vi "ResponseStringToSignalCluster(obj).vi"(8 "error in (no error)":errorcluster, 11 "T560Channel in":refnum<class "T560Channel.lvclass">) -> (0 "error out":errorcluster, 3 "T560Channel out":refnum<class "T560Channel.lvclass">)   [LabVIEW 2020, in "T560Channel.lvclass"]
doc: "Update the value of 'T560channel.Signal' cluster by converting the 'T560channel.Response' string"
uses:
  T560Channel.lvclass
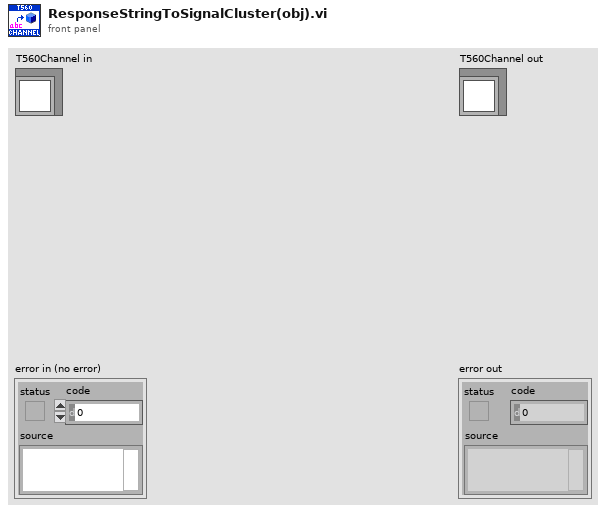
[diagram p1: front panel]
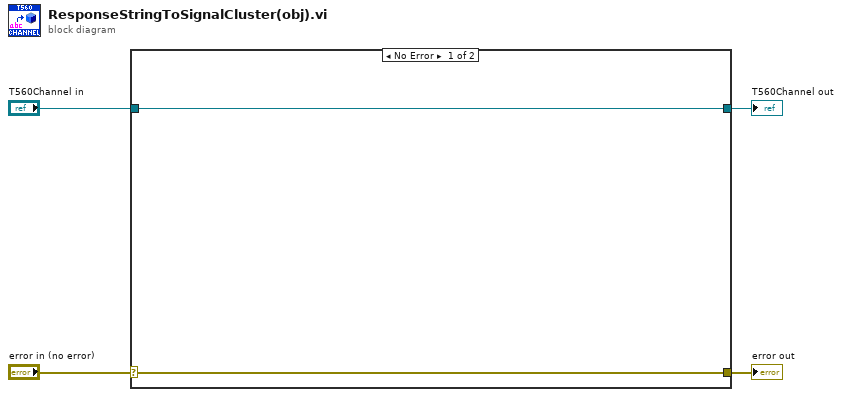
[diagram p0: block diagram]
diagram:
  n1 = case shown="No Error" "error in (no error)" {
    selector: "error in (no error)" -> [w6 w8]
    tunnel: [w6 w8] -> w3
    tunnel: [w5 w7] -> w1
    tunnel: "T560Channel in" -> [w5 w7]
    frame No Error {
    }
    frame Error {
    }
  }
  "error out" <- w3
  "T560Channel out" <- w1
